vi "Dequeue MHL Queue.vi"(8 "ErrorIn":errorcluster, 9 "Timeout(-1ms)":i32=-1) -> (0 "ErrorOut":errorcluster, 1 "Data":variant, 2 "Command":string)   [LabVIEW 2020, in "main.lvlib"]
doc: "Dequeue Element from MHL Queue"
uses:
  main.lvlib
  PTRL/QueueHandler/SubVis/Read.vi
  PTRL/QueueHandler/QueueHandler.lvlib
panel:
  # "Description\n\nDequeue Element from MHL Queue"
  # "INPUTS"
  # "OUTPUTS"
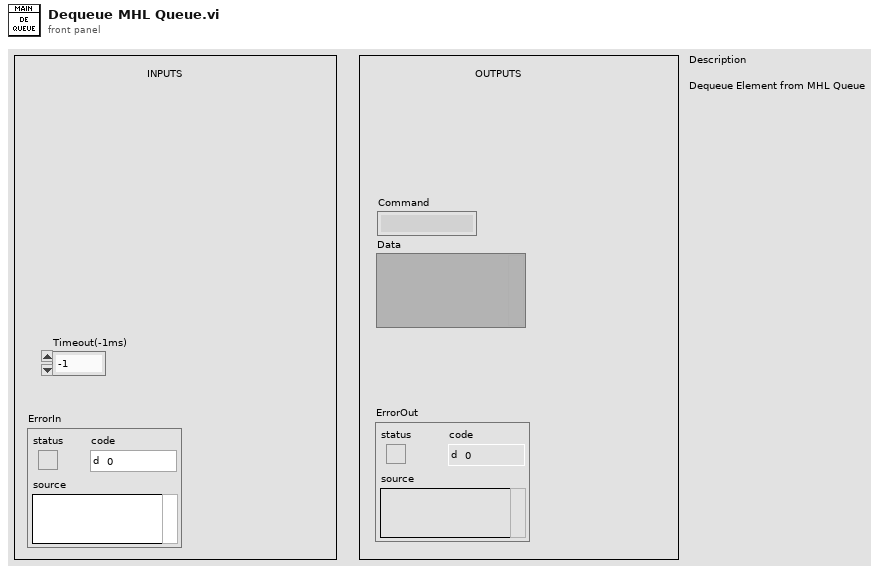
[diagram p1: front panel]
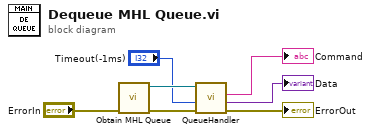
[diagram p0: block diagram]
diagram:
  n1 = call "Obtain MHL Queue.vi"("ErrorIn"="ErrorIn") -> ("ErrorOut"=w4:errorcluster, "MHL Queue Out"=w6:refnum<queue>)  [unwired: 9 in]
  n2 = call-poly "QueueHandler.vi"("ErrorIn"=w4, "Timeout(-1ms)"="Timeout(-1ms)", "MHL Queue In"=w6) -> ("ErrorOut"=→"ErrorOut":errorcluster, "Data"=→"Data":variant, "Command"=→"Command":string)  [unwired: 4 in, 2 out]
